vi "SetExternalInterfaces.vi"(8 "ErrorIn":errorcluster, 11 "ProgressQueue":refnum<queue>) -> (0 "ErrorOut":errorcluster)   [LabVIEW 2021, in "Application.lvclass"]
doc: "Sets the external interfaces of all ITAFObjects supported objects. This allows the object to communicate with the objects depends on"
uses:
  Application.lvclass
  Interface_TAF_IApplicationConfiguration/IApplicationConfiguration/IApplicationConfiguration.lvclass
  Interface_TAF_ITAFObject/ITAFObject/ITAFObject.lvclass
  5c5df808-c013-4a6b-85e3-bbe17662ba10.vi
  <vilib>/TriekselSoft/TracerLibrary/TracerLibrary/Tracer/protected/SendMessage.vi
  <vilib>/TriekselSoft/TracerLibrary/TracerLibrary/Tracer/protected/Timestamp.vi
  <vilib>/TriekselSoft/TracerLibrary/TracerLibrary/Tracer/Tracer_Level-Debug.vi
  <vilib>/TriekselSoft/TracerLibrary/TracerLibrary/Tracer/protected/Tracer_ClassAttributes.vi
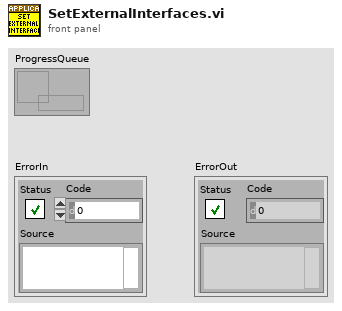
[diagram p1: front panel]
types:
  T1 = typedef "Application.lvclass/ObjectAttributes.ctl" = cluster{"Objects":variant, "BasePath":path, "Application":refnum<class "Application.lvclass">}
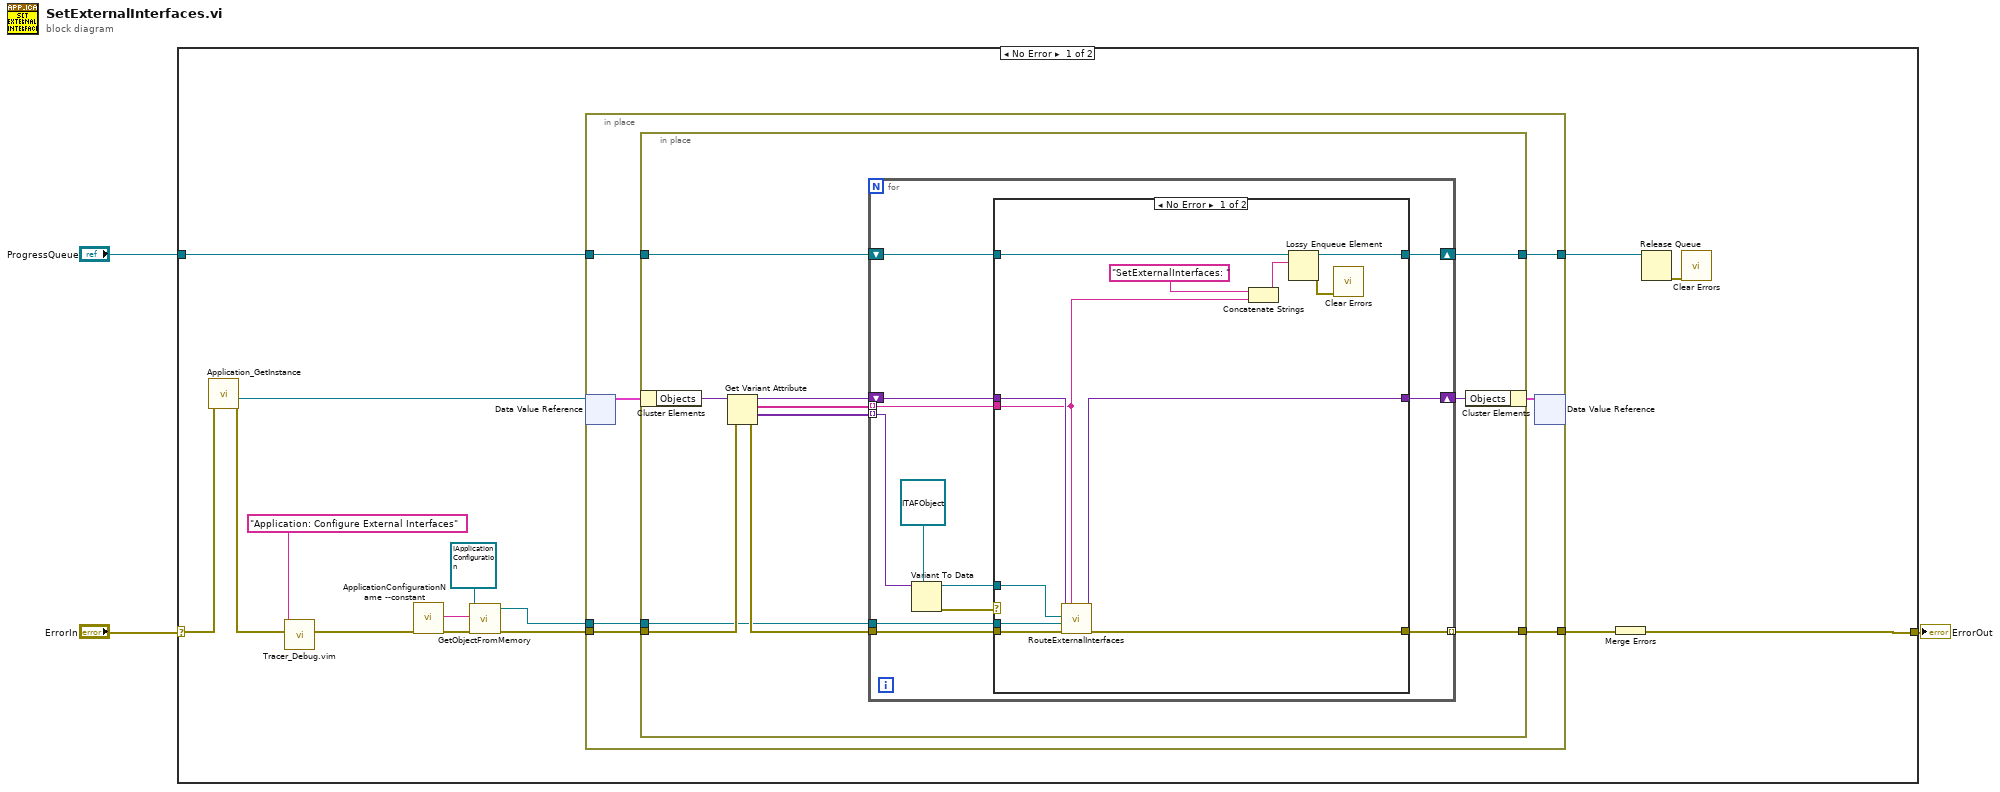
[diagram p0: block diagram]
diagram:
  n1 = case shown="No Error" "ErrorIn" {
    selector: "ErrorIn" -> [w16 w63]
    tunnel: [w14 w63] -> w2
    tunnel: "ProgressQueue" -> [w10 _]
    frame No Error {
      n2 = call "Application_GetInstance.vi"("ErrorIn"=w16) -> ("ErrorOut"=w15:errorcluster, "DVRRefOut"=w8:refnum<data-value>)  [unwired: 6 in, 3 out]
      n3 = call "Tracer_Debug.vim"("Error In"=w15, "Text"="Application: Configure External Interfaces") -> ("Error Out"=w13:errorcluster)  [unwired: 9 in]
      n4 = call "ApplicationConfigurationName --constant.vi"() -> ("AppConfigName"=w5:string)  [unwired: 10 in, 1 out]
      n5 = call "GetObjectFromMemory.vi"("ErrorIn"=w13, "ObjectName"=w5, "Type"=refnum<class "IApplicationConfiguration.lvclass"> refnum ("IApplicationStructure")) -> ("ErrorOut"=w12:errorcluster, "ObjectOut"=w4:refnum<class "IApplicationConfiguration.lvclass">)  [unwired: 7 in]
      n6 = in-place {
        in-place-border: w12 -> [w24]
        in-place-border: w10 -> [w23]
        in-place-border: [w22] -> w9
        in-place-border: [w19] -> w7
        in-place-border: w4 -> [w18]
        n7 = in-place-dvr #1(w8) -> (w21:T1)  [unwired: 1 out]
        n8 = in-place {
          in-place-border: w24 -> [w34]
          in-place-border: w23 -> [w33]
          in-place-border: [w32] -> w22
          in-place-border: [w26] -> w19
          in-place-border: w18 -> [w25]
          n9 = in-place-cluster #2(w21) -> ("Objects"=w30:variant)
          n10 = Get Variant Attribute(Variant=w30, error in=w34) -> (duplicate Variant=w29:variant, names=w27:string[], values=w28:variant[], error out=w35:errorcluster)  [unwired: 2 in]
          n11 = for {
            tunnel: w35 -> [w45]
            shift-right: [w43] -> w32
            shift-left: w33 -> [w44]
            shift-right: [w41] -> w31
            shift-left: w29 -> [w42]
            tunnel: w28 -> [w40] mode=indexing
            tunnel: w27 -> [w36] mode=indexing
            tunnel: [w46] -> w26 mode=indexing
            tunnel: w25 -> [w37]
            n12 = Variant To Data(type=refnum<class "ITAFObject.lvclass"> refnum ("NamedCreator"), Variant=w40) -> (data=w38:refnum<class "ITAFObject.lvclass">, error out=w47:errorcluster)  [unwired: 1 in]
            n13 = case shown="No Error" w47 {
              tunnel: w44 -> [w56 w61]
              tunnel: [w55 w61] -> w43
              tunnel: w42 -> [w50 w60]
              tunnel: [w54 w60] -> w41
              tunnel: w36 -> [w48 _]
              tunnel: w38 -> [w51 _]
              tunnel: [w58 w62] -> w46
              tunnel: w37 -> [w49 _]
              tunnel: w45 -> [w57 w62]
              frame No Error {
                n14 = call "RouteExternalInterfaces.vi"("ObjectName"=w48, "ErrorIn"=w57, "ConfigObject"=w49, "ITAFObjectIn"=w51, "VariantIn"=w50) -> ("ErrorOut"=w58:errorcluster, "VariantOut"=w54:variant)  [unwired: 5 in]
                n15 = Concatenate Strings("SetExternalInterfaces: " ("string"), w48) -> (w53:string)
                n16 = Lossy Enqueue Element(queue=w56, element=w53) -> (queue out=w55:refnum<queue>, error out=w59:errorcluster)  [unwired: 1 in, 2 out]
                n17 = call <vilib>:"Clear Errors.vi"("error in (no error)"=w59) -> ()  [unwired: 5 in, 2 out]
              }
              frame Error {
              }
            }
          }
          n18 = in-place-cluster #2("Objects"=w31) -> (w20:T1)
        }
        n19 = in-place-dvr #1(w20) -> ()  [unwired: 2 out]
      }
      n20 = Merge Errors(w7) -> (w14:errorcluster)
      n21 = Release Queue(queue=w9) -> (error out=w17:errorcluster)  [unwired: 2 in, 2 out]
      n22 = call <vilib>:"Clear Errors.vi"("error in (no error)"=w17) -> ()  [unwired: 5 in, 2 out]
    }
    frame Error {
    }
  }
  "ErrorOut" <- w2
